vi "MessageName.vi"() -> (2 "MessageName":string)   [LabVIEW 2020, in "TcpServerHello.lvlib"]
uses:
  TcpServerHello.lvlib
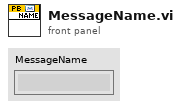
[diagram p1: front panel]
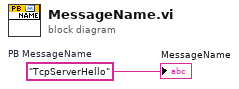
[diagram p0: block diagram]
diagram:
  w1 = "TcpServerHello"  # PB MessageName
  "MessageName" <- w1
